vi "Load Several Chirp Files.vi"   [LabVIEW 2012]
uses:
  LabVIEW/user.lib/SpectralRadar.llb/OCT Device.lvclass
  LabVIEW/user.lib/SpectralRadar.llb/Processing.lvclass
types:
  T1 = enum16{"Offset Errors", "Apodization Spectrum", "Apodization Vector", "Chirp", "Extended Adjust"}
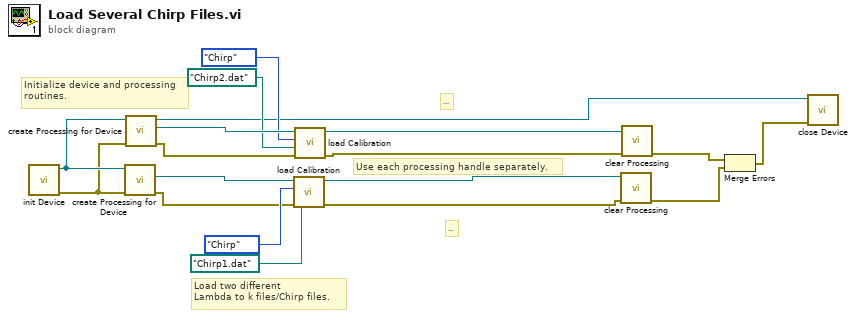
[diagram p0: block diagram]
diagram:
  # "..."
  # "..."
  # "Use each processing handle separately."
  # "Load two different \nLambda to k files/Chirp files."
  # "Initialize device and processing\nroutines."
  n1 = call "init Device.vi"() -> ("error out"=w17:errorcluster, "OCTDevice"=w18:refnum<class "OCT Device.lvclass">)  [unwired: 6 in]
  n2 = call "create Processing for Device.vi"("error in (no error)"=w17, "OCTDevice"=w18) -> ("error out"=w10:errorcluster, "Processing"=w14:refnum<class "Processing.lvclass">)  [unwired: 3 in, 1 out]
  n3 = call "create Processing for Device.vi"("error in (no error)"=w17, "OCTDevice"=w18) -> ("error out"=w9:errorcluster, "Processing"=w16:refnum<class "Processing.lvclass">, "OCTDevice"=w4:refnum<class "OCT Device.lvclass">)  [unwired: 3 in]
  n4 = call "load Calibration.vi"("error in (no error)"=w10, "Path"=path "Chirp1.dat", "Calibration Data"=T1."Chirp", "Processing"=w14) -> ("error out"=w6:errorcluster, "Processing"=w7:refnum<class "Processing.lvclass">)  [unwired: 2 in]
  n5 = call "load Calibration.vi"("error in (no error)"=w9, "Path"=path "Chirp2.dat", "Calibration Data"=T1."Chirp", "Processing"=w16) -> ("error out"=w5:errorcluster, "Processing"=w8:refnum<class "Processing.lvclass">)  [unwired: 2 in]
  n6 = call "clear Processing.vi"("error in (no error)"=w6, "Processing"=w7) -> ("error out"=w3:errorcluster)  [unwired: 5 in]
  n7 = call "clear Processing.vi"("error in (no error)"=w5, "Processing"=w8) -> ("error out"=w2:errorcluster)  [unwired: 5 in]
  n8 = Merge Errors(w2, w3) -> (w1:errorcluster)
  n9 = call "close Device.vi"("error in (no error)"=w1, "OCTDevice"=w4) -> ()  [unwired: 5 in, 1 out]
